vi "AdaptToInputs.vi"(3 "Term Types":T1[](array[typedef]), 4 "XRef":refnum<vi>, 5 "State In":T4={"Input Type"=variant(dbl 0.0), "Width"=0, "Typedef Name"="", "Value Type"=variant, "Selection"=0, "Options"=[], "Selections"=[], "Display Selections"=[], "Element Names"=[], "Typedef Name Width"=0, "Display Selection Width"=[], "Code Generated"=FALSE, "Is DVR"=FALSE, "Write Lock"=FALSE}) -> (0 "Reply":string[](array[string]), 2 "State Out":T4={"Input Type"=variant(dbl 0.0), "Width"=0, "Typedef Name"="", "Value Type"=variant, "Selection"=0, "Options"=[], "Selections"=[], "Display Selections"=[], "Element Names"=[], "Typedef Name Width"=0, "Display Selection Width"=[], "Code Generated"=FALSE, "Is DVR"=FALSE, "Write Lock"=FALSE})   [LabVIEW 2015, in "Read-Write-Signals.xnode"]
doc: "This ability VI is called by LabVIEW during type propagation so that your XNode may adapt itself to new input types. Term Types is an array of pairs of current Term IDs and the type descriptors corresponding to them. The type descriptors are taken from the signal connected to the terminal. Unwired terminals are not included in the array. Use Reply to inform LabVIEW of any actions it needs to take.\n\nDefault behavior: None.\n\nThis ability does not provide UI and OS messages are not handled."
uses:
  Read-Write-Signals.xnode
  State.ctl
  Read-Write-Signals Item.ctl
  Read-Write-Signals Sub Item.ctl
  Read-Write-Signals Sub Item Type.ctl
  Read-Write-Signals Selection.ctl
  Read-Write-Signals Display Selection.ctl
  <vilib>/XNodeSupport/XNodeTermTypeIDPair.ctl
  <vilib>/XNodeSupport/XNodeType.ctl
  <vilib>/XNodeSupport/XNodeString.ctl
  <vilib>/regexp/Match Regular Expression.xnode
  <vilib>/Erdos Miller/LV-Scripting/LV-Scripting.lvlib
  <vilib>/Utility/Data Type/NI_Data Type.lvlib
  <vilib>/XNodeSupport/NI_XNodeSupport.lvlib
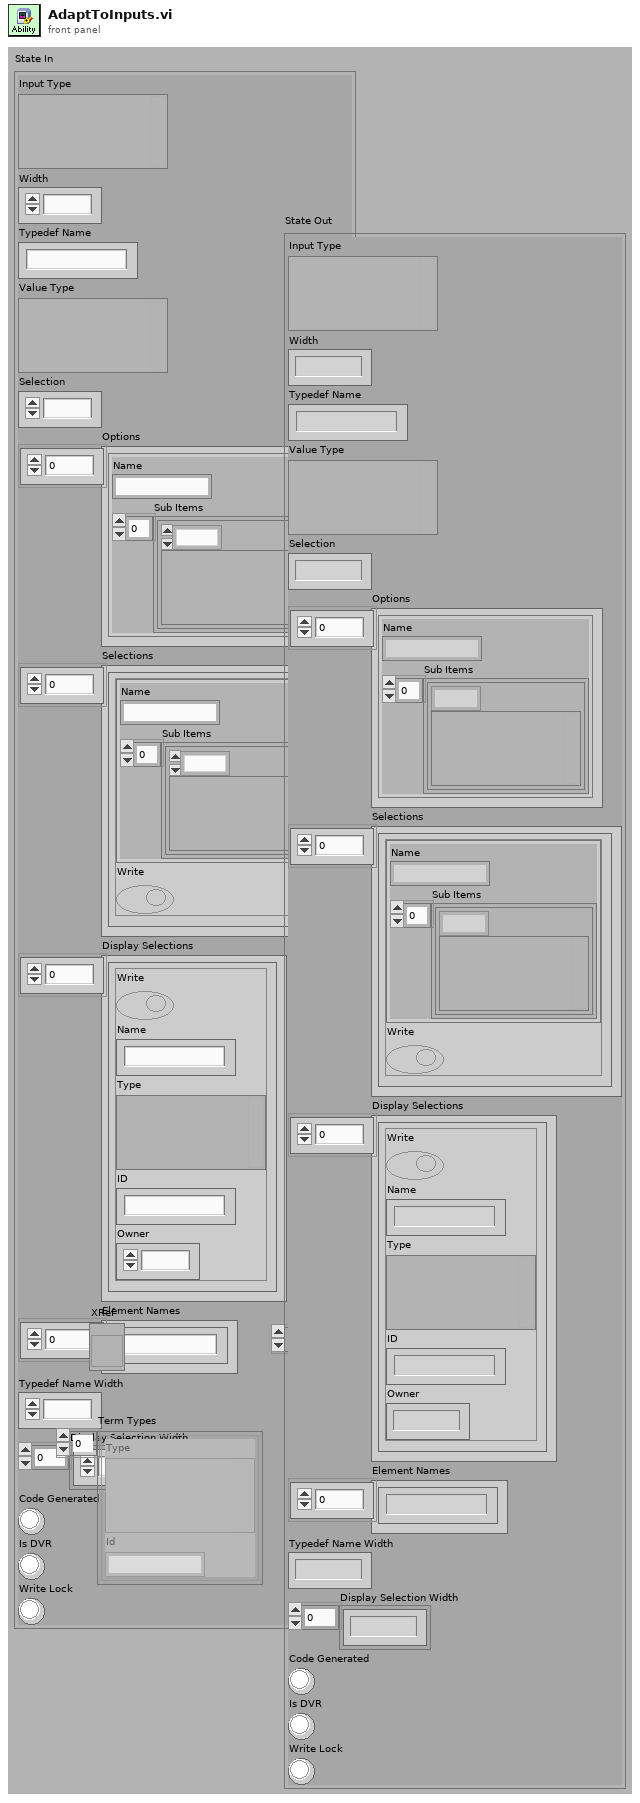
[diagram p1: front panel]
types:
  T1 = typedef "NI_XNodeSupport.lvlib/XNodeTermTypeIDPair.ctl" = cluster{"Type":T2, "Id":T3}
  T2 = typedef "NI_XNodeSupport.lvlib/XNodeType.ctl" = variant
  T3 = typedef "NI_XNodeSupport.lvlib/XNodeString.ctl" = string
  T4 = typedef "Read-Write-Signals.xnode/State.ctl" = cluster{"Input Type":variant, "Width":i32, "Typedef Name":string, "Value Type":variant, "Selection":i32, "Options":T5[], "Selections":T8[], "Display Selections":T9[], "Element Names":string[], "Typedef Name Width":i32, "Display Selection Width":i32[], "Code Generated":bool, "Is DVR":bool, "Write Lock":bool}
  T5 = typedef "Read-Write-Signals Item.ctl" = cluster{"Name":string, "Sub Items":T6[]}
  T6 = typedef "Read-Write-Signals Sub Item.ctl" = cluster{"Type":T7, "Value":variant}
  T7 = typedef "Read-Write-Signals Sub Item Type.ctl" = enum8{"Cluster Element", "Array Element", "Subarray"}
  T8 = typedef "Read-Write-Signals Selection.ctl" = cluster{"Item":T5, "Write":bool}
  T9 = typedef "Read-Write-Signals Display Selection.ctl" = cluster{"Write":bool, "Name":string, "Type":variant, "ID":string, "Owner":i32}
  T10 = typedef "NI_Data Type.lvlib/Refnum Type.ctl" = enum16{"NotARefnum", "UnknownRefnum", "Generic", "Datalog", "ByteStream", "Device", "Occurence", "TCPNetConnection", "Auto", "Menu", "Imaq", "Hardware", "DataSocket", "Visa", "IVI", "UDPNetConnection", "Notifier", "Queue", "Irda", "EventReg", "DotNet", "UserEvent", "Callback", "UNUSED_EMPTY_POSITION", "BlueToothNetConnection", "LVObjApp", "LVObjVI", "LVObjUnknown", "GenericClass", "UserDefinedRefnumTag", "DataValue", "RT FIFO", "TDMS File"}
  T11 = typedef "NI_Data Type.lvlib/Type Definition Info.ctl" = cluster{"Name":string, "Timestamp":u32}
  T12 = cluster{"Input Type":bool, "Width":bool, "Typedef Name":bool, "Value Type":bool, "Selection":bool, "Options":cluster{"Name":bool, "Sub Items":cluster{"Type":bool, "Value":bool}[]}[], "Selections":cluster{"Item":cluster{"Name":bool, "Sub Items":cluster{"Type":bool, "Value":bool}[]}, "Write":bool}[], "Display Selections":cluster{"Write":bool, "Name":bool, "Type":bool, "ID":bool, "Owner":bool}[], "Element Names":bool[], "Typedef Name Width":bool, "Display Selection Width":bool[], "Code Generated":bool, "Is DVR":bool, "Write Lock":bool}
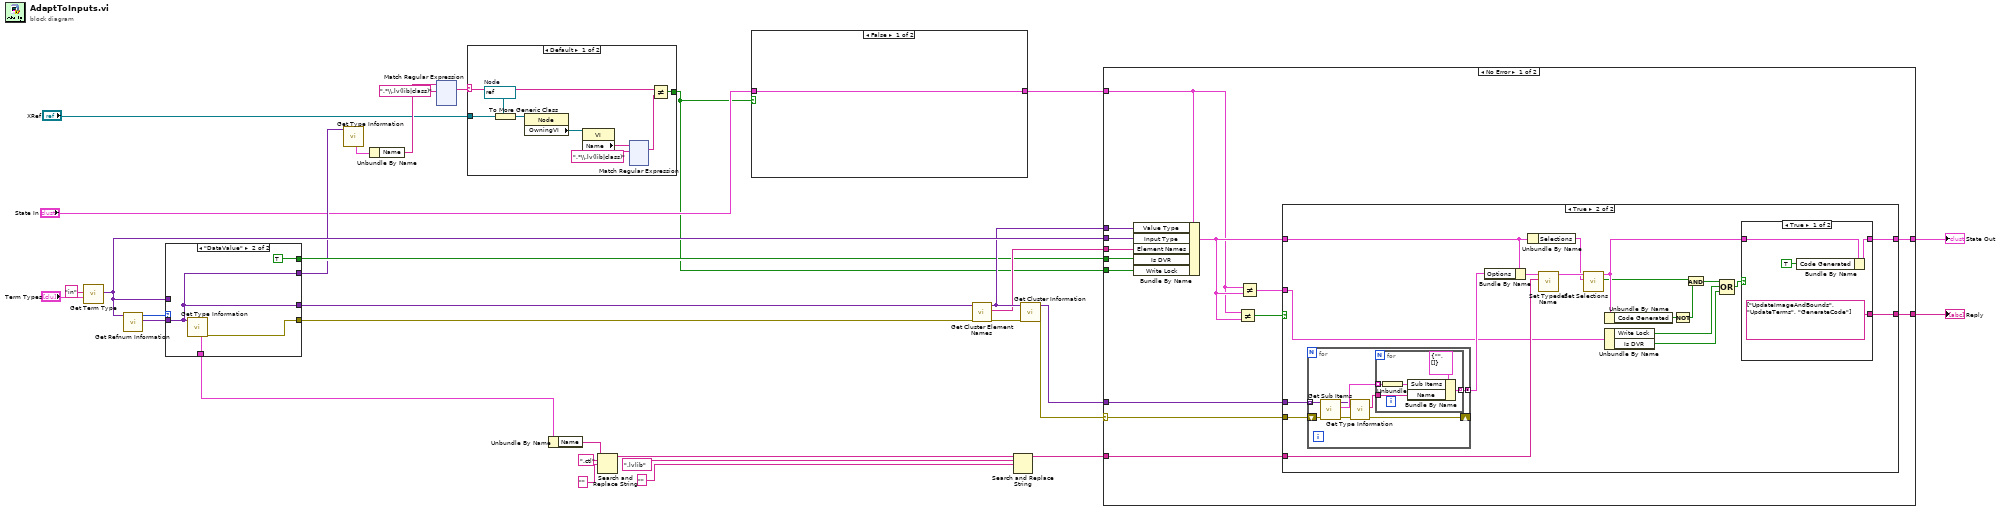
[diagram p0: block diagram]
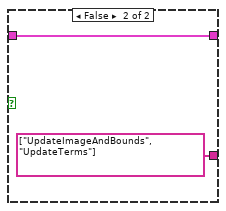
[diagram p3: hidden frame]
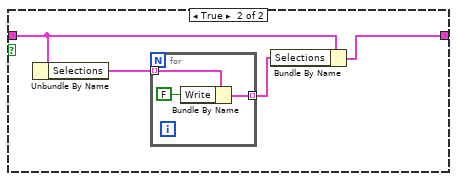
[diagram p5: hidden frame]
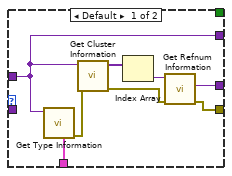
[diagram p6: hidden frame]
diagram:
  n1 = call <vilib>:"Get Term Type.vi"("Term Types"="Term Types", "ID"="in") -> ("Type"=w28:variant)  [unwired: 9 in]
  n2 = call <vilib>:"Get Refnum Information.vi"("Variant"=w28) -> ("Strict Type"=w6:variant, "Reference Type"=w7:T10)  [unwired: 7 in, 2 out]
  n3 = case shown="\"DataValue\"" w7 {
    tunnel: w28 -> [w33 _]
    tunnel: [w37 w44] -> w22
    tunnel: [w35 w43] -> w15
    tunnel: [w34 w41] -> w11
    tunnel: w6 -> [_ w41]
    tunnel: [_ TRUE] -> w5
    tunnel: [w33 w41] -> w4
    frame Default {
      n4 = call <vilib>:"Get Type Information.vi"("Variant"=w33) -> ("error out"=w36:errorcluster, "Type Definition Info"=w37:T11)  [unwired: 6 in, 3 out]
      n5 = call <vilib>:"Get Cluster Information.vi"("error in (no error)"=w36, "Variant"=w33) -> ("error out"=w38:errorcluster, "Cluster Elements"=w40:variant[])  [unwired: 8 in]
      n6 = Index Array(array=w40) -> (element=w39:variant)  [unwired: 1 in]
      n7 = call <vilib>:"Get Refnum Information.vi"("error in (no error)"=w38, "Variant"=w39) -> ("error out"=w35:errorcluster, "Strict Type"=w34:variant)  [unwired: 6 in, 2 out]
    }
    frame "DataValue" {
      n8 = call <vilib>:"Get Type Information.vi"("Variant"=w41) -> ("error out"=w43:errorcluster, "Type Definition Info"=w44:T11)  [unwired: 6 in, 3 out]
    }
  }
  n9 = call <vilib>:"Get Type Information.vi"("Variant"=w4) -> ("Type Definition Info"=w27:T11)  [unwired: 6 in, 4 out]
  n10 = Unbundle By Name(w27) -> ("Name"=w26:string)
  n11 = xnode "Match Regular Expression"("input string"=w26, "regular expression"=".*\\.lv(lib|class)") -> ("whole match"=w24:string)  [unwired: 4 in, 4 out]
  n12 = case shown="Default" w24 {
    selector: w24 -> [w46 _]
    tunnel: "XRef" -> [w53 _]
    tunnel: [w45 _] -> w1
    frame Default {
      w51 = refnum<vi> refnum  # Node
      n13 = To More Generic Class(target class=w51, reference=w53) -> (generic class reference=w52:refnum<vi>)
      n14 = property class="Node"(reference=w52) -> ("OwningVI"=w50:refnum<vi>)  [unwired: 1 in, 2 out]
      n15 = property class="VI"(reference=w50) -> ("Name"=w48:string)  [unwired: 1 in, 2 out]
      n16 = xnode "Match Regular Expression"("input string"=w48, "regular expression"=".*\\.lv(lib|class)") -> ("whole match"=w47:string)  [unwired: 4 in, 4 out]
      n17 = Not Equal?(x=w46, y=w47) -> (x != y?=w45:bool)
    }
    frame "" {
    }
  }
  n18 = Unbundle By Name(w22) -> ("Name"=w21:string)
  n19 = Search and Replace String(input string=w21, search string=".ctl", replace string="" ("search string")) -> (result string=w16:string)  [unwired: 5 in, 3 out]
  n20 = case shown="False" w1 {
    tunnel: "State In" -> [w168 w170]
    tunnel: [w168 w169] -> w3
    frame False {
    }
    frame True {
      n21 = Unbundle By Name(w170) -> ("Selections"=w172:T8[])
      n22 = for {
        tunnel: w172 -> [w175] mode=indexing
        tunnel: [w173] -> w171 mode=indexing
        n23 = Bundle By Name(cluster=w175, "Write"=FALSE) -> (w173:T8)
      }
      n24 = Bundle By Name(cluster=w170, "Selections"=w171) -> (w169:T4)
    }
  }
  n25 = call <vilib>:"Get Cluster Element Names.vi"("error in (no error)"=w15, "Cluster in"=w11) -> ("error out"=w12:errorcluster, "Names"=w9:string[], "Cluster  out"=w10:variant)  [unwired: 7 in]
  n26 = Search and Replace String(input string=w16, search string=".lvlib", replace string="" ("search string")) -> (result string=w13:string)  [unwired: 5 in, 3 out]
  n27 = call <vilib>:"Get Cluster Information.vi"("error in (no error)"=w12, "Variant"=w10) -> ("error out"=w8:errorcluster, "Cluster Elements"=w14:variant[])  [unwired: 8 in]
  n28 = case shown="No Error" w8 {
    selector: w8 -> [w182 _]
    tunnel: [w189 _] -> w30
    tunnel: [w188 w229] -> w29
    tunnel: w28 -> [w187 _]
    tunnel: w14 -> [w186 _]
    tunnel: w13 -> [w185 _]
    tunnel: w10 -> [w184 _]
    tunnel: w9 -> [w183 _]
    tunnel: w5 -> [w181 _]
    tunnel: w3 -> [w178 w229]
    tunnel: w1 -> [w176 _]
    frame No Error {
      n29 = Bundle By Name(cluster=w178, "Value Type"=w184, "Input Type"=w187, "Element Names"=w183, "Is DVR"=w181, "Write Lock"=w176) -> (w179:T4)
      n30 = Not Equal?(x=w178, y=w179) -> (x != y?=w180:bool)
      n31 = Not Equal?(x=w178, y=w179) -> (x != y?=w177:T12)
      n32 = case shown="True" w180 {
        tunnel: [_ w209] -> w189
        tunnel: w186 -> [_ w208]
        tunnel: w179 -> [w190 w202]
        tunnel: [w190 w196] -> w188
        tunnel: w182 -> [_ w206]
        tunnel: w185 -> [_ w203]
        tunnel: w177 -> [_ w193]
        frame False {
        }
        frame True {
          n33 = for {
            tunnel: w208 -> [w221] mode=indexing
            shift-right: [w223] -> _
            shift-left: w206 -> [w219]
            tunnel: [w217] -> w207 mode=concatenating
            n34 = call "Get Sub Items.vi"("error in (no error)"=w219, "Type in"=w221) -> ("error out"=w218:errorcluster, "Sub Items"=w222:cluster{"Sub Items":T6[]}[], "Type out"=w220:variant)  [unwired: 7 in]
            n35 = call <vilib>:"Get Type Information.vi"("error in (no error)"=w218, "Variant"=w220) -> ("error out"=w223:errorcluster, "Name"=w216:string)  [unwired: 5 in, 3 out]
            n36 = for {
              tunnel: w222 -> [w228] mode=indexing
              tunnel: w216 -> [w227]
              tunnel: [w225] -> w217 mode=indexing
              n37 = Unbundle(w228) -> ("Sub Items"=w224:T6[])
              n38 = Bundle By Name(cluster=T5 {"Name"="", "Sub Items"=[]} ("Item"), "Sub Items"=w224, "Name"=w227) -> (w225:T5)
            }
          }
          n39 = Bundle By Name(cluster=w202, "Options"=w207) -> (w204:T4)
          n40 = Unbundle By Name(w202) -> ("Selections"=w201:T8[])
          n41 = call "Set Typedef Name.vi"("Typedef Name"=w203, "State in"=w204) -> ("State out"=w205:T4)  [unwired: 9 in]
          n42 = call "Set Selections.vi"("Selections"=w201, "State in"=w205) -> ("All Valid"=w197:bool, "State out"=w199:T4)  [unwired: 8 in]
          n43 = Unbundle By Name(w199) -> ("Code Generated"=w200:bool)
          n44 = Unbundle By Name(w193) -> ("Write Lock"=w192:bool, "Is DVR"=w191:bool)
          n45 = Not(x=w200) -> (.not. x?=w198:bool)
          n46 = And(x=w197, y=w198) -> (x .and. y?=w195:bool)
          n47 = Compound Arithmetic op=OR(w195, w192, w191) -> (w194:bool)
          n48 = case shown="True" w194 {
            tunnel: [string[] ["UpdateImageAndBounds", "UpdateTerms", "GenerateCode"] ("Reply") string[] ["UpdateImageAndBounds", "UpdateTerms"] ("Reply")] -> w209
            tunnel: w199 -> [w212 w214]
            tunnel: [w211 w214] -> w196
            frame True {
              n49 = Bundle By Name(cluster=w212, "Code Generated"=TRUE) -> (w211:T4)
            }
            frame False {
            }
          }
        }
      }
    }
    frame Error {
    }
  }
  "Reply" <- w30
  "State Out" <- w29
